vi "InitializeGrid.vi"(9 "n vertical":dbl, 10 "n horizontal":dbl, 11 "grid in":T1) -> (3 "grid out":T1)   [LabVIEW 2016]
uses:
  grid.ctl
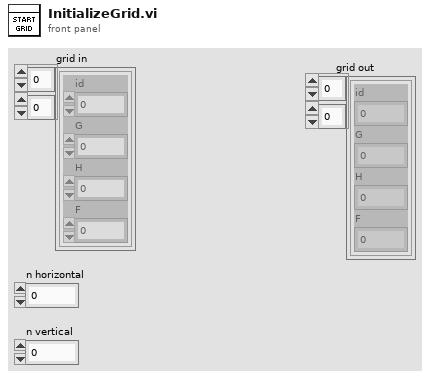
[diagram p1: front panel]
types:
  T1 = typedef "grid.ctl" = cluster{"id":dbl, "G":dbl, "H":dbl, "F":dbl}[][]
  T2 = cluster{"[0]":dbl, "[1]":dbl, "[2]":dbl, "[3]":dbl}
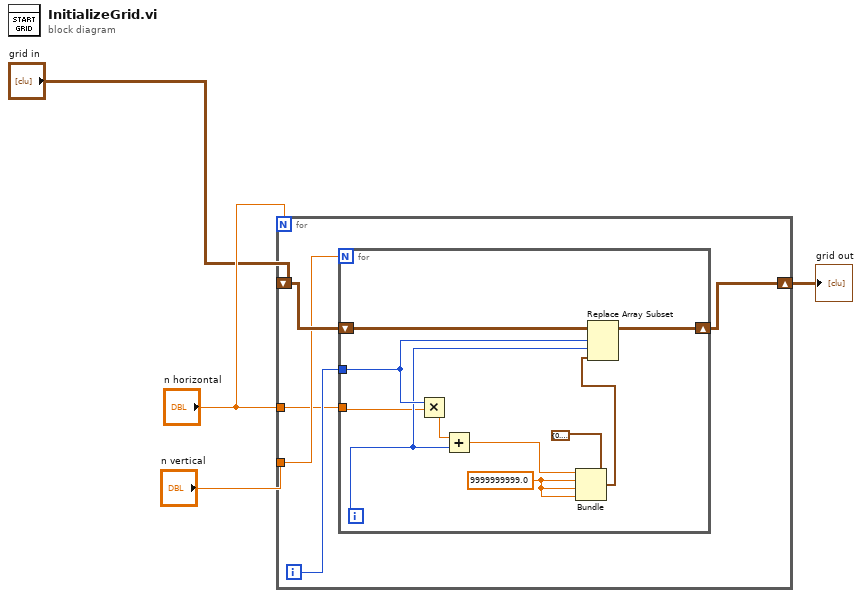
[diagram p0: block diagram]
diagram:
  n1 = for {
    N: "n horizontal" -> [_]
    shift-right: [w7] -> w1
    shift-left: "grid in" -> [w9]
    tunnel: "n vertical" -> [w6]
    tunnel: "n horizontal" -> [w5]
    i -> [w8]
    n2 = for {
      N: w6 -> [_]
      shift-right: [w14] -> w7
      shift-left: w9 -> [w16]
      tunnel: w8 -> [w15]
      tunnel: w5 -> [w11]
      i -> [w13]
      w10 = 9999999999.0
      n3 = Multiply(x=w15, y=w11) -> (x*y=w19:dbl)
      n4 = Add(x=w19, y=w13) -> (x+y=w17:dbl)
      n5 = Bundle(cluster=T2 {"[0]"=0.0, "[1]"=0.0, "[2]"=0.0, "[3]"=0.0} ("element 2"), "[0]"=w17, "[1]"=w10, "[2]"=w10, "[3]"=w10) -> (w12:T2)
      n6 = Replace Array Subset(array=w16, new element=w12, index (row)=w15, index (col)=w13) -> (w14:T1)
    }
  }
  "grid out" <- w1
